vi "Practica 11.vi"() -> ()   [LabVIEW 2018]
uses:
  <vilib>/LabVIEW Interface for Arduino/Type Defs/Board Type.ctl
  <vilib>/LabVIEW Interface for Arduino/LabVIEW Interface for Arduino.lvlib
panel:
  in  "Cerrar Puerto":bool
  in  "Valor de 0 a 255":dbl(slide) scale=0.0..255.0
  # "Practica 11: Control Salida Analógica"
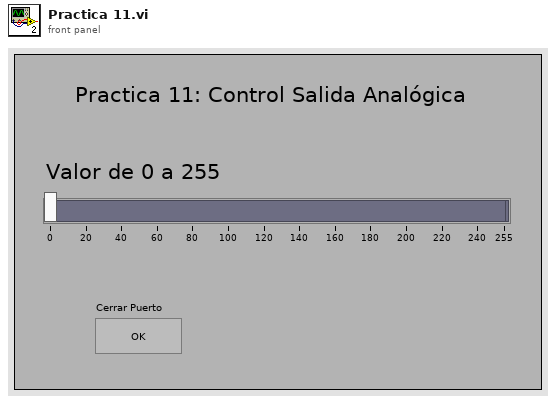
[diagram p1: front panel]
types:
  T1 = typedef "LabVIEW Interface for Arduino.lvlib/Board Type.ctl" = enum16{"Uno", "Dimuelanove w/Atmega 328", "Mega 2560"}
  T2 = typedef "LabVIEW Interface for Arduino.lvlib/Arduino Resource.ctl" = cluster{"VISA resource":refnum<visa-resource-name>, "Board Type":T1, "Connection Type":enum8{"USB / Serial"}, "Bytes Per Packet (15)":u8}
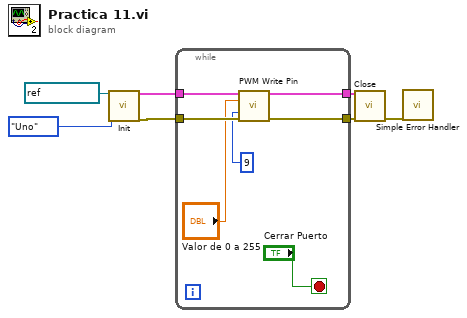
[diagram p0: block diagram]
diagram:
  n1 = call <vilib>:"Init.vi"("VISA resource"=refnum<visa-resource-name> "COM9", "Board Type (Uno)"=Board_Type."Uno") -> ("Arduino Resource"=w7:T2, "error out"=w6:errorcluster)  [unwired: 16 in]
  n2 = while {
    tunnel: w7 -> [w13]
    tunnel: w6 -> [w12]
    tunnel: [w11] -> w5
    tunnel: [w10] -> w4
    stop <- "Cerrar Puerto" stop-if-true
    n3 = call <vilib>:"PWM Write Pin.vi"("Arduino Resource"=w13, "Duty Cycle (0 - 255)"="Valor de 0 a 255", "PWM Pin (3)"=u8 9, "error in"=w12) -> ("Arduino Resource"=w11:T2, "error out"=w10:errorcluster)  [unwired: 10 in]
  }
  n4 = call <vilib>:"Close.vi"("Arduino Resource"=w5, "error in"=w4) -> ("error out"=w3:errorcluster)  [unwired: 13 in]
  n5 = call <vilib>:"Simple Error Handler.vi"("error in (no error)"=w3) -> ()  [unwired: 4 in, 5 out]
